vi "2_Button_change.vi"(6 "Unit of change":u8, 9 "Position in":u8, 10 "Decrement":bool, 11 "Increment":bool) -> (2 "Position out":u8, 3 "Update?":bool)   [LabVIEW 2012, in "Mecanum Drive.lvrbt"]
uses:
  Mecanum Drive.lvrbt
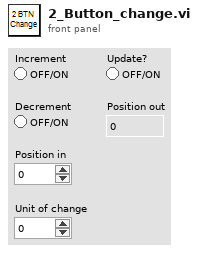
[diagram p1: front panel]
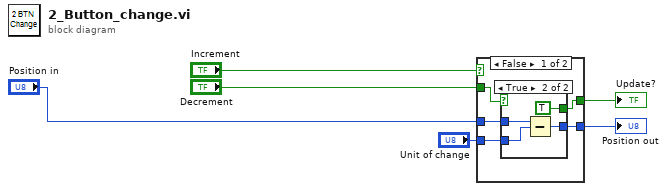
[diagram p0: block diagram]
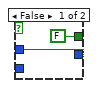
[diagram p2: hidden frame]
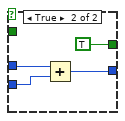
[diagram p3: hidden frame]
diagram:
  n1 = case shown="False" "Increment" {
    tunnel: "Decrement" -> [w11 _]
    tunnel: "Position in" -> [w10 w21]
    tunnel: [w9 w20] -> w4
    tunnel: [w8 TRUE] -> w5
    tunnel: "Unit of change" -> [w7 w18]
    frame False {
      n2 = case shown="True" w11 {
        tunnel: w10 -> [w13 w17]
        tunnel: [w13 w16] -> w9
        tunnel: [FALSE TRUE] -> w8
        tunnel: w7 -> [_ w14]
        frame False {
        }
        frame True {
          n3 = Subtract(x=w17, y=w14) -> (x-y=w16:u8)
        }
      }
    }
    frame True {
      n4 = Add(x=w21, y=w18) -> (x+y=w20:u8)
    }
  }
  "Update?" <- w5
  "Position out" <- w4
